vi "Load Commands.vi"(6 "Constants":refnum<class "Sequence Constants.lvclass">, 8 "error in":refnum<class "MultiErrors.lvclass">, 10 "Config Element":refnum<class "Config Element.lvclass">) -> (0 "error out":refnum<class "MultiErrors.lvclass">, 2 "Commands":refnum<class "Command Config.lvclass">[](array[class]))   [LabVIEW 2020, in "VolatusSeqConfig.lvlib" / "Sequence Config.lvclass"]
uses:
  Sequence Config.lvclass
  lv-cdm/CDM-Config/Config Element/Config Element.lvclass
  Command Config/Command Config.lvclass
  VolatusErrorUtilities/MultiErrors/MultiErrors.lvclass
  VolatusErrorUtilities/MultiErrors/MultiErrors.lvclass/MultiErrors.ctl
  Command Type.ctl
  Sequence Config.lvclass/Sequence Config.ctl
  VolatusSeqConfig.lvlib
  Sequence Constants/Sequence Constants.lvclass
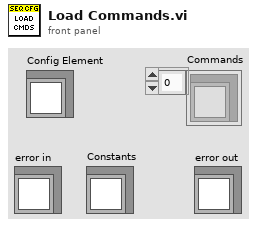
[diagram p1: front panel]
types:
  T1 = typedef "VolatusSeqConfig.lvlib/Command Type.ctl" = enum16{"Digital", "Numeric", "Transition", "Stop", "StartLog", "StopLog", "Start", "Event", "Error", "HTTP"}
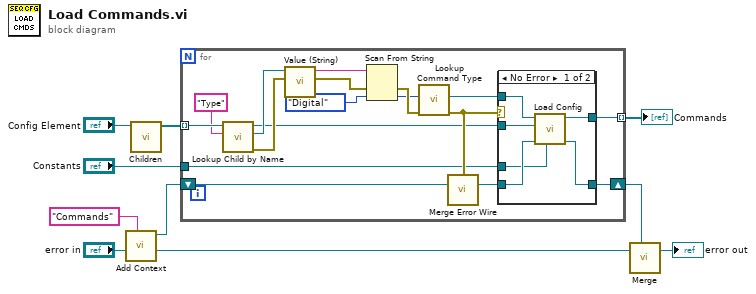
[diagram p0: block diagram]
diagram:
  n1 = call "Add Context.vi"("Context"="Commands", "MultiErrors in"="error in") -> ("Original Context"=w3:refnum<class "MultiErrors.lvclass">, "Added Context"=w5:refnum<class "MultiErrors.lvclass">)  [unwired: 8 in]
  n2 = call "Children.vi"("Config Element in"="Config Element") -> ("Elements"=w9:refnum<class "Config Element.lvclass">[])  [unwired: 9 in, 1 out]
  n3 = for {
    tunnel: w9 -> [w24] mode=indexing
    tunnel: [w19] -> w8 mode=indexing
    shift-right: [w16] -> w4
    shift-left: w5 -> [w18]
    tunnel: "Constants" -> [w11]
    n4 = call "Lookup Child by Name.vi"("Name"="Type", "Config Element in"=w24) -> ("error out"=w26:errorcluster, "Child"=w22:refnum<class "Config Element.lvclass">, "Config Element out"=w20:refnum<class "Config Element.lvclass">)  [unwired: 6 in, 1 out]
    n5 = call "Value (String).vi"("error in (no error)"=w26, "Config Element in"=w22) -> ("error out"=w14:errorcluster, "String Value"=w15:string)  [unwired: 8 in]
    n6 = Scan From String(input string=w15, error in=w14, default 1=Command_Type."Digital" ("Command Type")) -> (error out=w27:errorcluster, output 1=w12:T1)  [unwired: 2 in, 2 out]
    n7 = call "Lookup Command Type.vi"("error in (no error)"=w27, "Command Type"=w12) -> ("error out"=w25:errorcluster, "Command"=w21:refnum<class "Command Config.lvclass">)  [unwired: 8 in]
    n8 = call "Merge Error Wire.vi"("error in (no error)"=w25, "MultiErrors in"=w18) -> ("MultiErrors out"=w17:refnum<class "MultiErrors.lvclass">)  [unwired: 13 in]
    n9 = case shown="No Error" w25 {
      tunnel: w21 -> [w33 _]
      tunnel: w20 -> [w32 _]
      tunnel: [w31 _] -> w19
      tunnel: w17 -> [w30 w34]
      tunnel: [w29 w34] -> w16
      tunnel: w11 -> [w28 _]
      frame No Error {
        n10 = call-dynamic "Load Config.vi"("Constants"=w28, "error in (no error)"=w30, "Config Element"=w32, "Command Config in"=w33) -> ("error out"=w29:refnum<class "MultiErrors.lvclass">, "Command Config out"=w31:refnum<class "Command Config.lvclass">)  [unwired: 6 in]
      }
      frame Error {
      }
    }
  }
  "Commands" <- w8
  n11 = call "Merge.vi"("First Error In"=w3, "Second Error In"=w4) -> ("MultiErrors out"=→"error out":refnum<class "MultiErrors.lvclass">)  [unwired: 5 in]
